vi "Washing Machine Problem (200 lit. Tank).vi"() -> ()   [LabVIEW 2016]
panel:
  out "Thermometer":dbl(slide) scale=0.0..100.0
  out "Tank":dbl(slide) scale=0.0..200.0
  out "Motor":bool
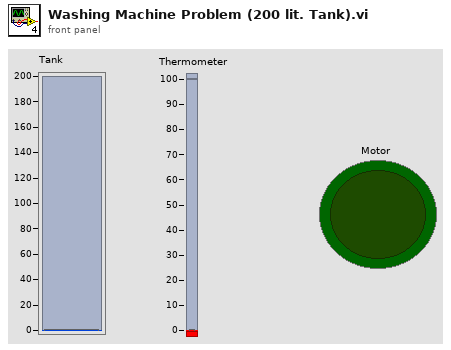
[diagram p1: front panel]
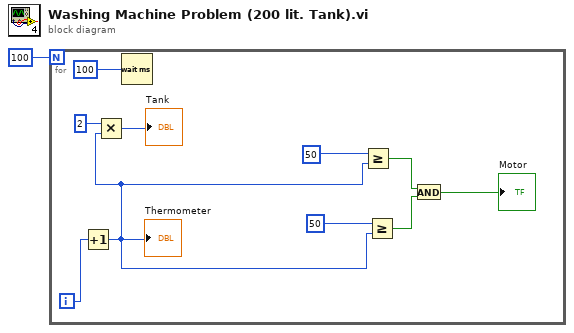
[diagram p0: block diagram]
diagram:
  n1 = for {
    N: 100 ("Numeric") -> [_]
    i -> [w11]
    n2 = Increment(x=w11) -> (x+1=w3:i32)
    "Thermometer" <- w3
    n3 = Multiply(x=2, y=w3) -> (x*y=→"Tank":i32)
    n4 = Wait (ms)(milliseconds to wait=100) -> ()  [unwired: 1 out]
    n5 = Greater Or Equal?(x=50, y=w3) -> (x >= y?=w7:bool)
    n6 = Greater Or Equal?(x=50, y=w3) -> (x >= y?=w8:bool)
    n7 = And(x=w7, y=w8) -> (x .and. y?=→"Motor":bool)
  }
